vi "SubSystems.vi"(8 "error in":errorcluster) -> ()   [LabVIEW 2019]
doc: "This VI calls the various robot subsystems that will then run in parallel. New subSystems will automatlically script code to make the call."
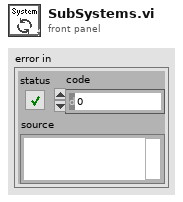
[diagram p1: front panel]
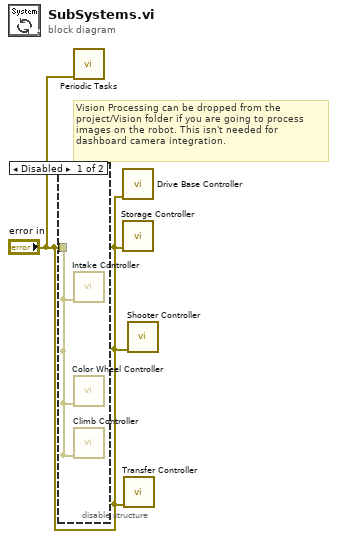
[diagram p0: block diagram]
diagram:
  # "Vision Processing can be dropped from the\nproject/Vision folder if you are going to process\nimages on the robot. This isn't needed for\ndashboard camera integration."
  n1 = disable-structure shown="Disabled" {
    disable-tunnel: "error in" -> [w2 _]
    frame Disabled {
      n2 = call "Intake Controller.vi"("error in"=w2) -> ()  [unwired: 11 in]
      n3 = call "Color Wheel Controller.vi"("error in"=w2) -> ()  [unwired: 11 in]
      n4 = call "Climb Controller.vi"("error in"=w2) -> ()  [unwired: 11 in]
    }
    frame Enabled {
    }
  }
  n5 = call "Periodic Tasks.vi"("error in"="error in") -> ()  [unwired: 1 in, 10 out]
  n6 = call "Drive Base Controller.vi"("error in"="error in") -> ()  [unwired: 11 in]
  n7 = call "Storage Controller.vi"("error in"="error in") -> ()  [unwired: 11 in]
  n8 = call "Transfer Controller.vi"("error in"="error in") -> ()  [unwired: 11 in]
  n9 = call "Shooter Controller.vi"("error in"="error in") -> ()  [unwired: 11 in]
